vi "IO.vi"() -> ()   [LabVIEW 2020]
uses:
  Global_Variable/Global.vi
  Libraries/S7/S7.lvlib
panel:
  in  "选项卡控件":enum32{"DI", "DO", "伺服"}(tab)
  out "I 1":T1
  out "I 3":T2
  out "I 2":T3
  out "I 0":T4
  out "I 4":T5
  out "I 5":T6
  in  "Q5":T6
  in  "Q4":T7
  in  "Q3":T8
  in  "Q2":T9
  in  "Q1":T10
  in  "Q0":T11
  in  "输入轴旋转手动速度":sgl caption="手动速度" format="%#.3f"
  in  "输入轴旋转-正转":bool
  in  "输入轴旋转-反转":bool
  in  "输入轴旋转绝对位置":sgl caption="绝对位置" format="%#.3f"
  in  "输入轴旋转相对位置":sgl caption="相对位置" format="%#.3f"
  out "输入轴旋转当前位置":sgl caption="当前位置" format="%#.3f"
  in  "输入轴旋转-绝对定位":bool
  in  "输入轴旋转-相对定位":bool
  in  "输入轴移载手动速度":sgl caption="手动速度" format="%#.3f"
  in  "输入轴移载-正转":bool
  in  "输入轴移载-反转":bool
  in  "输入轴移载绝对位置":sgl caption="绝对位置" format="%#.3f"
  in  "输入轴移载相对位置":sgl caption="相对位置" format="%#.3f"
  out "输入轴移载当前位置":sgl caption="当前位置" format="%#.3f"
  in  "输入轴移载-绝对定位":bool
  in  "输入轴移载-相对定位":bool
  in  "工装移载手动速度":sgl caption="手动速度" format="%#.3f"
  in  "工装移载-正转":bool
  in  "工装移载-反转":bool
  in  "工装移载绝对位置":sgl caption="绝对位置" format="%#.3f"
  in  "工装移载相对位置":sgl caption="相对位置" format="%#.3f"
  out "工装移载当前位置":sgl caption="当前位置" format="%#.3f"
  in  "工装移载-绝对定位":bool
  in  "工装移载-相对定位":bool
  out "输入轴旋转状态":bool
  out "输入轴移载状态":bool
  out "工装移载状态":bool
  out "输出轴旋转状态":bool
  out "输入扭矩":sgl format="%#.3f"
  out "输出扭矩(小)":sgl format="%#.3f"
  out "输出扭矩(大)":sgl format="%#.3f"
  out "吸收电流":sgl format="%#.3f"
  # "手动操作"
  # "输入轴旋转伺服"
  # "输入轴移载伺服"
  # "工装移载伺服"
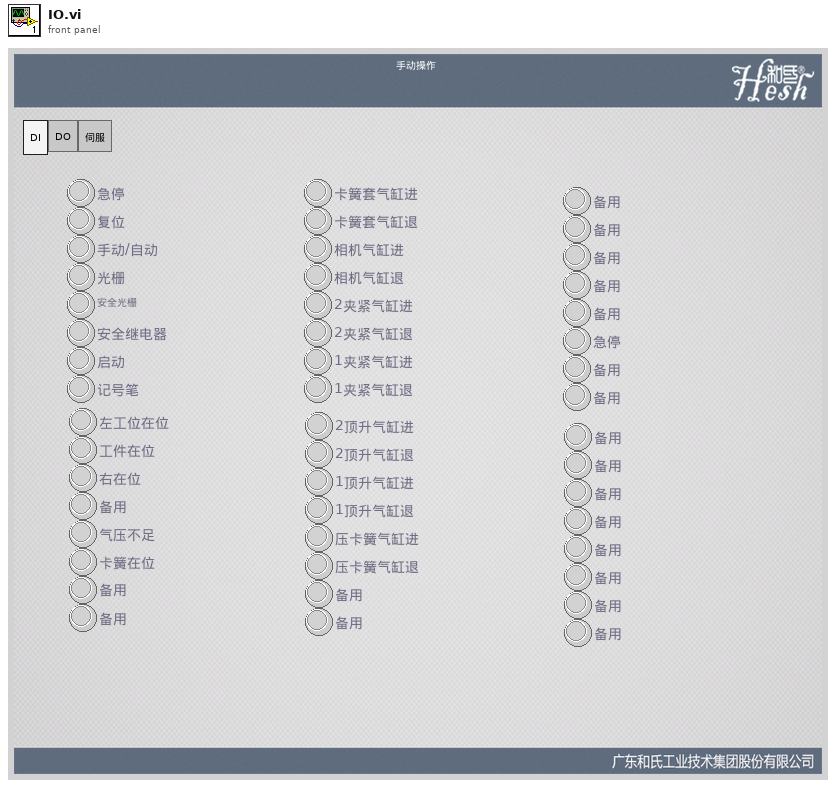
[diagram p1: front panel]
types:
  T1 = cluster{"左工位在位":bool, "工件在位":bool, "右在位":bool, "备用":bool, "气压不足":bool, "卡簧在位":bool, "备用":bool, "备用 ":bool}
  T2 = cluster{"2顶升气缸进":bool, "2顶升气缸退":bool, "1顶升气缸进":bool, "1顶升气缸退":bool, "压卡簧气缸进":bool, "压卡簧气缸退":bool, "备用":bool, "备用":bool}
  T3 = cluster{"卡簧套气缸进":bool, "卡簧套气缸退":bool, "相机气缸进":bool, "相机气缸退":bool, "2夹紧气缸进":bool, "2夹紧气缸退":bool, "1夹紧气缸进":bool, "1夹紧气缸退":bool}
  T4 = cluster{"急停":bool, "复位":bool, "手动/自动":bool, "光栅":bool, "安全光栅":bool, "安全继电器":bool, "启动":bool, "记号笔":bool}
  T5 = cluster{"备用":bool, "备用":bool, "备用":bool, "备用":bool, "备用":bool, "急停":bool, "备用":bool, "备用":bool}
  T6 = cluster{"备用":bool, "备用":bool, "备用":bool, "备用":bool, "备用":bool, "备用":bool, "备用":bool, "备用":bool}
  T7 = cluster{"总气源":bool, "3工位扶正气缸张开":bool, "备用":bool, "备用":bool, "备用":bool, "备用":bool, "备用":bool, "备用":bool}
  T8 = cluster{"2工位扶正气缸张开":bool, "2工位扶正气缸夹紧":bool, "2工位油缸前进":bool, "2工位抬升气缸升":bool, "3工位油缸进":bool, "2工位抬升气缸降":bool, "2工位增压切换":bool, "3工位扶正气缸夹紧":bool}
  T9 = cluster{"1工位轴承上料气缸进":bool, "1工位轴承上料气缸退":bool, "1工位轴承顶升气缸升":bool, "1工位轴承顶升气缸降":bool, "2工位定型气缸进":bool, "2工位定型气缸退":bool, "3工位旋转气缸进":bool, "3工位旋转气缸退":bool}
  T10 = cluster{"OK指示":bool, "NG指示":bool, "/":bool, "/":bool, "/":bool, "/":bool, "/":bool, "/":bool}
  T11 = cluster{"备用":bool, "备用":bool, "备用":bool, "备用":bool, "蜂鸣器":bool, "三色灯黄":bool, "三色灯绿":bool, "三色灯红":bool}
  T12 = cluster{bool, bool, bool, bool, bool, bool, bool, bool}
  T13 = cluster{"[0]":bool, "[1]":bool, "[2]":bool, "[3]":bool, "[4]":bool, "[5]":bool, "[6]":bool, "[7]":bool}
  T14 = typedef "S7.lvlib/Read_Data (Reply Payload)--cluster.ctl" = cluster{"读取成功":bool, "数据":u32[], "Read_Data_error":errorcluster}
  T15 = cluster{"Boolean array[0]":bool, "Boolean array[1]":bool, "Boolean array[2]":bool, "Boolean array[3]":bool, "Boolean array[4]":bool, "Boolean array[5]":bool, "Boolean array[6]":bool, "Boolean array[7]":bool}
  T16 = cluster{"电缸压力":dbl, "电缸位移":sgl, "工装移载位移":sgl, "1":sgl, "输入扭矩":sgl, "大幅":sgl, "输出扭矩(大)":sgl, "大幅度":sgl}
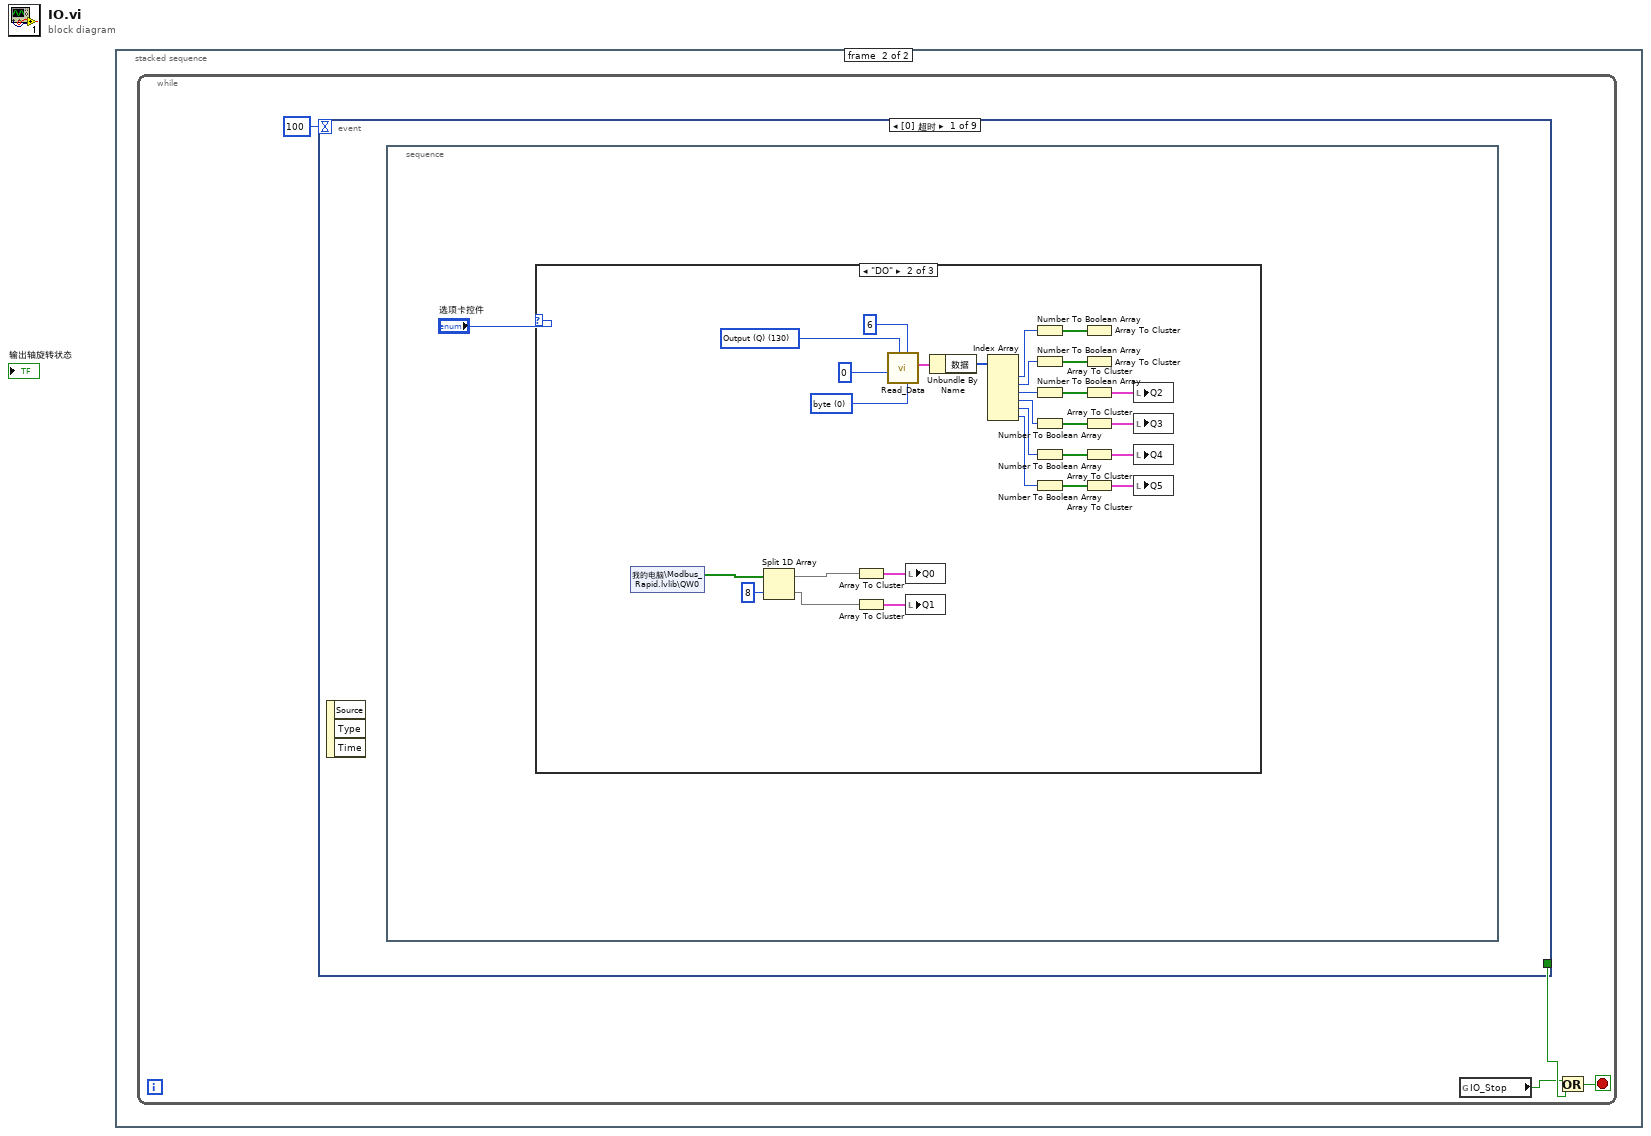
[diagram p0: block diagram]
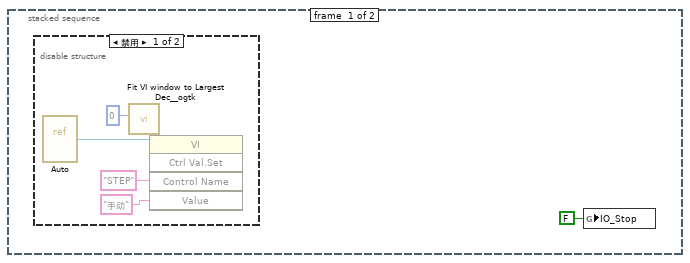
[diagram p2: hidden frame]
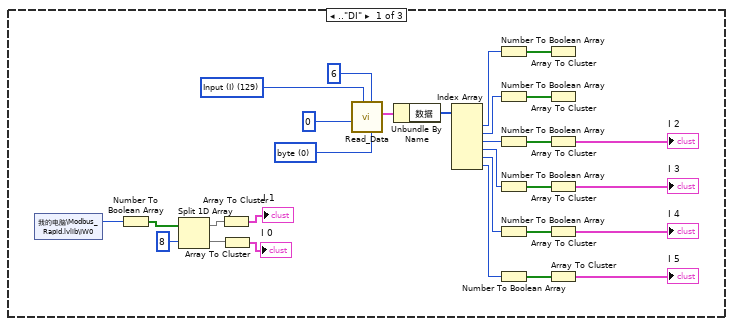
[diagram p4: hidden frame]
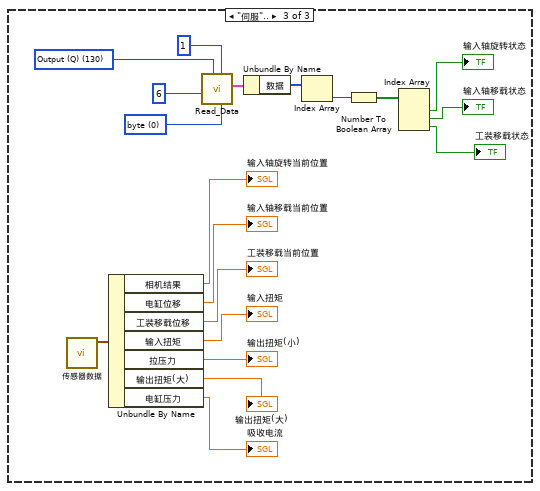
[diagram p5: hidden frame]
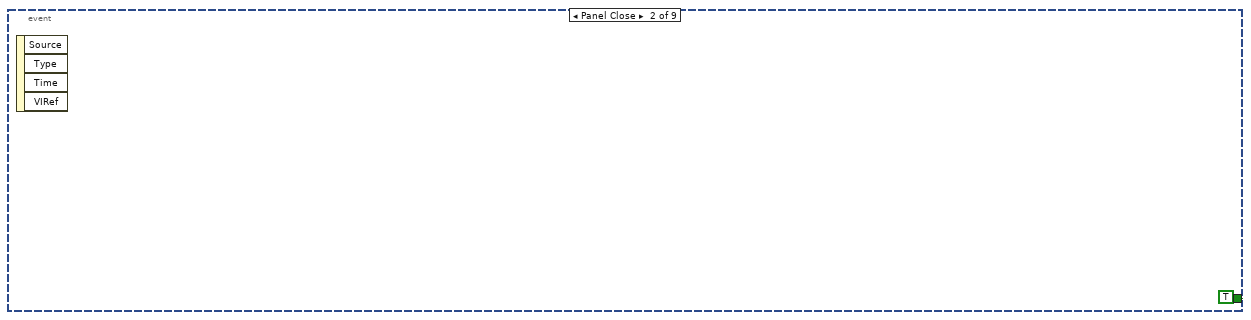
[diagram p6: hidden frame]
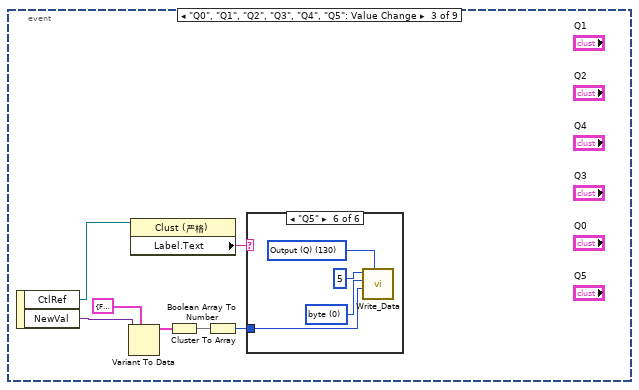
[diagram p7: hidden frame]
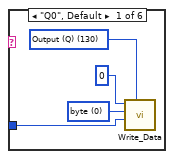
[diagram p8: hidden frame]
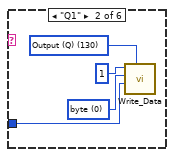
[diagram p9: hidden frame]
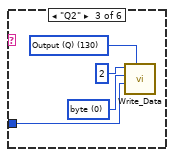
[diagram p10: hidden frame]
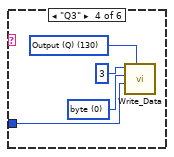
[diagram p11: hidden frame]
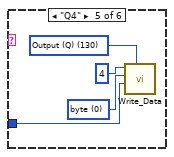
[diagram p12: hidden frame]
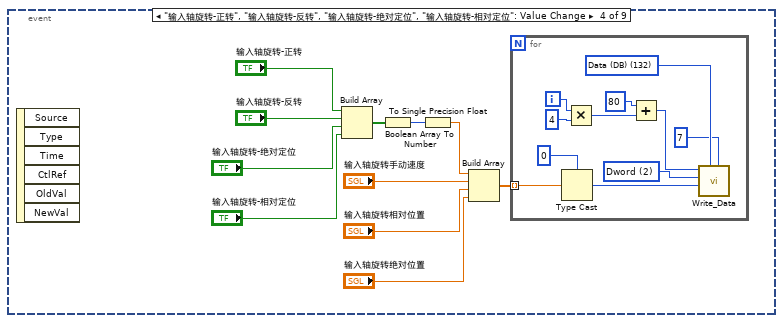
[diagram p13: hidden frame]
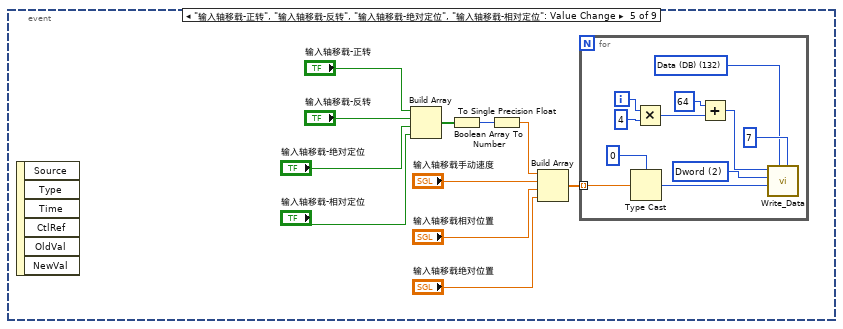
[diagram p14: hidden frame]
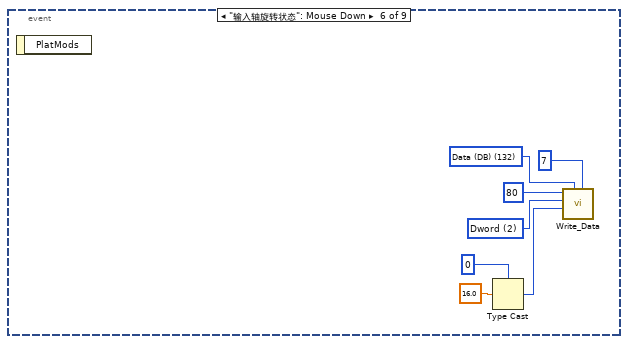
[diagram p15: hidden frame]
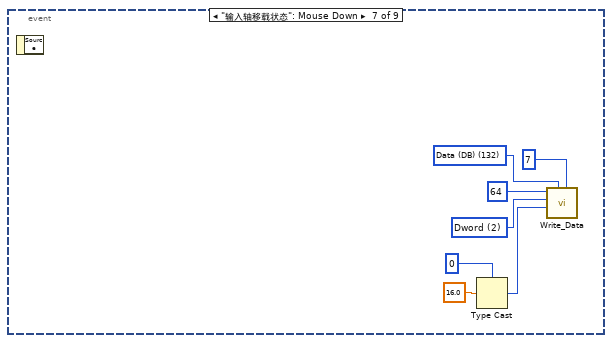
[diagram p16: hidden frame]
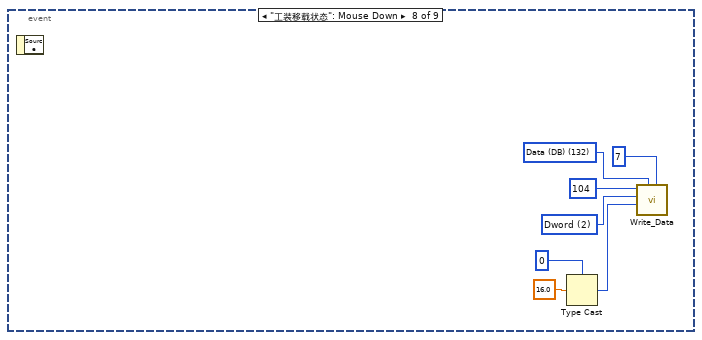
[diagram p17: hidden frame]
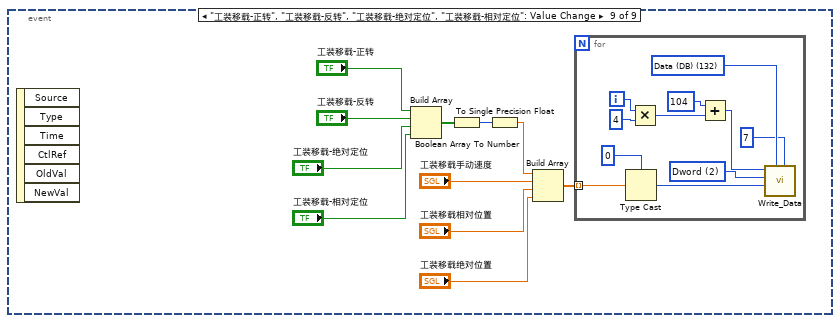
[diagram p18: hidden frame]
diagram:
  n1 = stacked-sequence {
    frame #0 {
      n2 = disable-structure shown="禁用" {
        frame Disabled {
          n3 = vi-ref "Auto.vi"() -> (w4:refnum<vi>)
          n4 = call <userlib>:"Fit VI window to Largest Dec__ogtk.vi"("border spacing (2 px)"=0) -> ()  [unwired: 5 in, 2 out]
          n5 = invoke class="VI" method="Ctrl Val.Set"(reference=w4, "Control Name"="STEP" ("控件名"), "Value"="手动" ("控件名")) -> ()  [unwired: 2 in, 5 out]
        }
        frame Enabled {
        }
      }
      n6 = global write "Global.vi" "IO_Stop"(FALSE ("IO_Stop")) -> ()
    }
    frame #1 {
      n7 = while {
        stop <- w6 stop-if-true
        n8 = event shown="[0] 超时" {
          selector: _ -> [_ _ _ _ _ _ _ _ _]
          dyn-events: _ -> [_ _ _ _ _ _ _ _ _]
          timeout: 100 -> [_ _ _ _ _ _ _ _ _]
          tunnel: [_ TRUE _ _ _ _ _ _ _] -> w8
          event Timeout {
            n9 = event-data() -> ()  [unwired: 1 in, 3 out]
            n10 = stacked-sequence {
              frame #0 {
                n11 = case shown="\"DO\"" "选项卡控件" {
                  frame .."DI" {
                    w21 = u16 0 items=["byte", "word", "Dword"] ("数据类型")
                    w19 = u8 129 items=["I/O (P)"=128, "Input (I)"=129, "Output (Q)"=130, "Bit Memory (M)"=131, "Data (DB)"=132, "Instance Data (DI)"=133, "Local Data (L)"=134, "Predecessor Local Data (VL)"=135] ("寄存器类型")
                    n12 = shared-variable "我的电脑\\Modbus_Rapid.lvlib\\IW0"() -> (w17:u16)  [unwired: 1 in, 1 out]
                    n13 = Number To Boolean Array(number=w17) -> (Boolean array=w16:bool[])
                    n14 = Split 1D Array(array=w16, index=8 ("索引")) -> (first subarray=w15:bool[], second subarray=w13:bool[])
                    n15 = Array To Cluster(array=w15) -> (cluster=→"I 1":T13)
                    n16 = Array To Cluster(array=w13) -> (cluster=→"I 0":T13)
                    n17 = call "Read_Data.vi"("数据类型"=w21, "读取长度"=u16 6, "寄存器类型"=w19, "起始地址"=u32 0) -> ("Reply Payload"=w23:T14)  [unwired: 5 in, 2 out]
                    n18 = Unbundle By Name(w23) -> ("数据"=w22:u32[])
                    n19 = Index Array(array=w22) -> (element #1=w35:u32, element #2=w37:u32, element #3=w36:u32, element #4=w32:u32, element #5=w31:u32, element #6=w30:u32)  [unwired: 6 in]
                    n20 = Number To Boolean Array(number=w35) -> (Boolean array=w34:bool[])
                    n21 = Number To Boolean Array(number=w37) -> (Boolean array=w33:bool[])
                    n22 = Number To Boolean Array(number=w36) -> (Boolean array=w29:bool[])
                    n23 = Number To Boolean Array(number=w32) -> (Boolean array=w27:bool[])
                    n24 = Number To Boolean Array(number=w31) -> (Boolean array=w25:bool[])
                    n25 = Number To Boolean Array(number=w30) -> (Boolean array=w24:bool[])
                    n26 = Array To Cluster(array=w34) -> ()  [unwired: 1 out]
                    n27 = Array To Cluster(array=w33) -> ()  [unwired: 1 out]
                    n28 = Array To Cluster(array=w29) -> (cluster=→"I 2":T15)
                    n29 = Array To Cluster(array=w27) -> (cluster=→"I 3":T15)
                    n30 = Array To Cluster(array=w25) -> (cluster=→"I 4":T15)
                    n31 = Array To Cluster(array=w24) -> (cluster=→"I 5":T15)
                  }
                  frame "DO" {
                    w49 = u16 0 items=["byte", "word", "Dword"] ("数据类型")
                    w47 = u8 130 items=["I/O (P)"=128, "Input (I)"=129, "Output (Q)"=130, "Bit Memory (M)"=131, "Data (DB)"=132, "Instance Data (DI)"=133, "Local Data (L)"=134, "Predecessor Local Data (VL)"=135] ("寄存器类型")
                    n32 = shared-variable "我的电脑\\Modbus_Rapid.lvlib\\QW0"() -> (w40:bool[])  [unwired: 1 in, 1 out]
                    n33 = Split 1D Array(array=w40, index=8 ("索引")) -> (first subarray=w42:bool[], second subarray=w41:bool[])
                    n34 = Array To Cluster(array=w42) -> (cluster=w44:T13)
                    n35 = Array To Cluster(array=w41) -> (cluster=w43:T13)
                    n36 = call "Read_Data.vi"("数据类型"=w49, "读取长度"=u16 6, "寄存器类型"=w47, "起始地址"=u32 0) -> ("Reply Payload"=w66:T14)  [unwired: 5 in, 2 out]
                    n37 = local write "Q0"(w44) -> ()
                    n38 = local write "Q1"(w43) -> ()
                    n39 = Unbundle By Name(w66) -> ("数据"=w67:u32[])
                    n40 = Index Array(array=w67) -> (element #1=w57:u32, element #2=w59:u32, element #3=w58:u32, element #4=w56:u32, element #5=w55:u32, element #6=w54:u32)  [unwired: 6 in]
                    n41 = Number To Boolean Array(number=w57) -> (Boolean array=w60:bool[])
                    n42 = Number To Boolean Array(number=w59) -> (Boolean array=w61:bool[])
                    n43 = Number To Boolean Array(number=w58) -> (Boolean array=w62:bool[])
                    n44 = Number To Boolean Array(number=w56) -> (Boolean array=w63:bool[])
                    n45 = Number To Boolean Array(number=w55) -> (Boolean array=w64:bool[])
                    n46 = Number To Boolean Array(number=w54) -> (Boolean array=w65:bool[])
                    n47 = Array To Cluster(array=w60) -> ()  [unwired: 1 out]
                    n48 = Array To Cluster(array=w61) -> ()  [unwired: 1 out]
                    n49 = Array To Cluster(array=w62) -> (cluster=w52:T15)
                    n50 = Array To Cluster(array=w63) -> (cluster=w53:T15)
                    n51 = Array To Cluster(array=w64) -> (cluster=w51:T15)
                    n52 = Array To Cluster(array=w65) -> (cluster=w50:T15)
                    n53 = local write "Q2"(w52) -> ()
                    n54 = local write "Q3"(w53) -> ()
                    n55 = local write "Q4"(w51) -> ()
                    n56 = local write "Q5"(w50) -> ()
                  }
                  frame "伺服".. {
                    w79 = u16 0 items=["byte", "word", "Dword"] ("数据类型")
                    w77 = u8 130 items=["I/O (P)"=128, "Input (I)"=129, "Output (Q)"=130, "Bit Memory (M)"=131, "Data (DB)"=132, "Instance Data (DI)"=133, "Local Data (L)"=134, "Predecessor Local Data (VL)"=135] ("寄存器类型")
                    n57 = call "传感器数据.vi"() -> ("传感器读数"=w71:T16)  [unwired: 11 in]
                    n58 = Unbundle By Name(w71) -> ("相机结果"=→"输入轴旋转当前位置":dbl, "电缸位移"=→"输入轴移载当前位置":sgl, "工装移载位移"=→"工装移载当前位置":sgl, "输入扭矩"=→"输入扭矩":sgl, "拉压力"=→"输出扭矩(小)":sgl, "输出扭矩(大)"=→"输出扭矩(大)":sgl, "电缸压力"=→"吸收电流":dbl)
                    n59 = call "Read_Data.vi"("数据类型"=w79, "读取长度"=u16 1, "寄存器类型"=w77, "起始地址"=u32 6) -> ("Reply Payload"=w80:T14)  [unwired: 5 in, 2 out]
                    n60 = Unbundle By Name(w80) -> ("数据"=w81:u32[])
                    n61 = Index Array(array=w81) -> (element=w86:u32)  [unwired: 1 in]
                    n62 = Number To Boolean Array(number=w86) -> (Boolean array=w83:bool[])
                    n63 = Index Array(array=w83) -> (element #1=→"输入轴旋转状态":bool, element #2=→"输入轴移载状态":bool, element #3=→"工装移载状态":bool)  [unwired: 3 in]
                  }
                }
              }
            }
          }
          event Panel Close {
            n64 = event-data() -> ()  [unwired: 1 in, 4 out]
          }
          event "Q0", "Q1", "Q2", "Q3", "Q4", "Q5": Value Change {
            n65 = event-data() -> ("CtlRef"=w89:refnum<vi>, "NewVal"=w93:variant)  [unwired: 1 in]
            n66 = Variant To Data(type=T12 {FALSE, FALSE, FALSE, FALSE, FALSE, FALSE, FALSE, FALSE}, Variant=w93) -> (data=w92:T12)  [unwired: 1 in, 1 out]
            n67 = property class="Clust (严格)"(reference=w89) -> ("Label.Text"=w88:string)  [unwired: 1 in, 2 out]
            n68 = Cluster To Array(cluster=w92) -> (array=w91:bool[])
            n69 = Boolean Array To Number(Boolean array=w91) -> (number=w90:u32)
            n70 = case shown="\"Q5\"" w88 {
              tunnel: w90 -> [w98 w102 w106 w110 w114 w118]
              frame "Q0", Default {
                w96 = u16 0 items=["byte", "word", "Dword"] ("数据类型")
                w97 = u8 130 items=["I/O (P)"=128, "Input (I)"=129, "Output (Q)"=130, "Bit Memory (M)"=131, "Data (DB)"=132, "Instance Data (DI)"=133, "Local Data (L)"=134, "Predecessor Local Data (VL)"=135] ("寄存器类型")
                n71 = call "Write_Data.vi"("寄存器类型"=w97, "写入数据"=w98, "数据类型"=w96, "写入地址"=u32 0) -> ()  [unwired: 5 in, 3 out]
              }
              frame "Q1" {
                w100 = u16 0 items=["byte", "word", "Dword"] ("数据类型")
                w101 = u8 130 items=["I/O (P)"=128, "Input (I)"=129, "Output (Q)"=130, "Bit Memory (M)"=131, "Data (DB)"=132, "Instance Data (DI)"=133, "Local Data (L)"=134, "Predecessor Local Data (VL)"=135] ("寄存器类型")
                n72 = call "Write_Data.vi"("寄存器类型"=w101, "写入数据"=w102, "数据类型"=w100, "写入地址"=u32 1) -> ()  [unwired: 5 in, 3 out]
              }
              frame "Q2" {
                w104 = u16 0 items=["byte", "word", "Dword"] ("数据类型")
                w105 = u8 130 items=["I/O (P)"=128, "Input (I)"=129, "Output (Q)"=130, "Bit Memory (M)"=131, "Data (DB)"=132, "Instance Data (DI)"=133, "Local Data (L)"=134, "Predecessor Local Data (VL)"=135] ("寄存器类型")
                n73 = call "Write_Data.vi"("寄存器类型"=w105, "写入数据"=w106, "数据类型"=w104, "写入地址"=u32 2) -> ()  [unwired: 5 in, 3 out]
              }
              frame "Q3" {
                w108 = u16 0 items=["byte", "word", "Dword"] ("数据类型")
                w109 = u8 130 items=["I/O (P)"=128, "Input (I)"=129, "Output (Q)"=130, "Bit Memory (M)"=131, "Data (DB)"=132, "Instance Data (DI)"=133, "Local Data (L)"=134, "Predecessor Local Data (VL)"=135] ("寄存器类型")
                n74 = call "Write_Data.vi"("寄存器类型"=w109, "写入数据"=w110, "数据类型"=w108, "写入地址"=u32 3) -> ()  [unwired: 5 in, 3 out]
              }
              frame "Q4" {
                w112 = u16 0 items=["byte", "word", "Dword"] ("数据类型")
                w113 = u8 130 items=["I/O (P)"=128, "Input (I)"=129, "Output (Q)"=130, "Bit Memory (M)"=131, "Data (DB)"=132, "Instance Data (DI)"=133, "Local Data (L)"=134, "Predecessor Local Data (VL)"=135] ("寄存器类型")
                n75 = call "Write_Data.vi"("寄存器类型"=w113, "写入数据"=w114, "数据类型"=w112, "写入地址"=u32 4) -> ()  [unwired: 5 in, 3 out]
              }
              frame "Q5" {
                w116 = u16 0 items=["byte", "word", "Dword"] ("数据类型")
                w117 = u8 130 items=["I/O (P)"=128, "Input (I)"=129, "Output (Q)"=130, "Bit Memory (M)"=131, "Data (DB)"=132, "Instance Data (DI)"=133, "Local Data (L)"=134, "Predecessor Local Data (VL)"=135] ("寄存器类型")
                n76 = call "Write_Data.vi"("寄存器类型"=w117, "写入数据"=w118, "数据类型"=w116, "写入地址"=u32 5) -> ()  [unwired: 5 in, 3 out]
              }
            }
          }
          event "输入轴旋转-正转", "输入轴旋转-反转", "输入轴旋转-绝对定位", "输入轴旋转-相对定位": Value Change {
            n77 = event-data() -> ()  [unwired: 1 in, 6 out]
            n78 = Build Array("输入轴旋转-正转", "输入轴旋转-反转", "输入轴旋转-绝对定位", "输入轴旋转-相对定位") -> (w128:bool[])
            n79 = Boolean Array To Number(Boolean array=w128) -> (number=w127:u32)
            n80 = To Single Precision Float(number=w127) -> (single precision float=w129:sgl)
            n81 = Build Array(w129, "输入轴旋转手动速度", "输入轴旋转相对位置", "输入轴旋转绝对位置") -> (w126:sgl[])
            n82 = for {
              tunnel: w126 -> [w135] mode=indexing
              i -> [w132]
              w137 = u16 2 items=["byte", "word", "Dword"] ("数据类型")
              w140 = u8 132 items=["I/O (P)"=128, "Input (I)"=129, "Output (Q)"=130, "Bit Memory (M)"=131, "Data (DB)"=132, "Instance Data (DI)"=133, "Local Data (L)"=134, "Predecessor Local Data (VL)"=135] ("寄存器类型")
              n83 = Type Cast(type=u32 0, x=w135) -> (*(type *) &x=w134:u32)
              n84 = Multiply(x=w132, y=u32 4) -> (x*y=w131:u32)
              n85 = Add(x=u32 80 ("写入地址"), y=w131) -> (x+y=w130:u32)
              n86 = call "Write_Data.vi"("DB #"=u16 7, "寄存器类型"=w140, "写入数据"=w134, "数据类型"=w137, "写入地址"=w130) -> ()  [unwired: 4 in, 3 out]
            }
          }
          event "输入轴移载-正转", "输入轴移载-反转", "输入轴移载-绝对定位", "输入轴移载-相对定位": Value Change {
            n87 = event-data() -> ()  [unwired: 1 in, 6 out]
            n88 = Build Array("输入轴移载-正转", "输入轴移载-反转", "输入轴移载-绝对定位", "输入轴移载-相对定位") -> (w150:bool[])
            n89 = Boolean Array To Number(Boolean array=w150) -> (number=w149:u32)
            n90 = To Single Precision Float(number=w149) -> (single precision float=w151:sgl)
            n91 = Build Array(w151, "输入轴移载手动速度", "输入轴移载相对位置", "输入轴移载绝对位置") -> (w148:sgl[])
            n92 = for {
              tunnel: w148 -> [w160] mode=indexing
              i -> [w158]
              w153 = u16 2 items=["byte", "word", "Dword"] ("数据类型")
              w155 = u8 132 items=["I/O (P)"=128, "Input (I)"=129, "Output (Q)"=130, "Bit Memory (M)"=131, "Data (DB)"=132, "Instance Data (DI)"=133, "Local Data (L)"=134, "Predecessor Local Data (VL)"=135] ("寄存器类型")
              n93 = Type Cast(type=u32 0, x=w160) -> (*(type *) &x=w152:u32)
              n94 = Multiply(x=w158, y=u32 4) -> (x*y=w157:u32)
              n95 = Add(x=u32 64 ("写入地址"), y=w157) -> (x+y=w154:u32)
              n96 = call "Write_Data.vi"("DB #"=u16 7, "寄存器类型"=w155, "写入数据"=w152, "数据类型"=w153, "写入地址"=w154) -> ()  [unwired: 4 in, 3 out]
            }
          }
          event "输入轴旋转状态": Mouse Down {
            w165 = u16 2 items=["byte", "word", "Dword"] ("数据类型")
            w167 = u8 132 items=["I/O (P)"=128, "Input (I)"=129, "Output (Q)"=130, "Bit Memory (M)"=131, "Data (DB)"=132, "Instance Data (DI)"=133, "Local Data (L)"=134, "Predecessor Local Data (VL)"=135] ("寄存器类型")
            n97 = event-data() -> ()  [unwired: 1 in, 1 out]
            n98 = Type Cast(type=u32 0, x=sgl 16.0) -> (*(type *) &x=w169:u32)
            n99 = call "Write_Data.vi"("DB #"=u16 7, "寄存器类型"=w167, "写入数据"=w169, "数据类型"=w165, "写入地址"=u32 80) -> ()  [unwired: 4 in, 3 out]
          }
          event "输入轴移载状态": Mouse Down {
            w170 = u16 2 items=["byte", "word", "Dword"] ("数据类型")
            w173 = u8 132 items=["I/O (P)"=128, "Input (I)"=129, "Output (Q)"=130, "Bit Memory (M)"=131, "Data (DB)"=132, "Instance Data (DI)"=133, "Local Data (L)"=134, "Predecessor Local Data (VL)"=135] ("寄存器类型")
            n100 = event-data() -> ()  [unwired: 1 in, 1 out]
            n101 = Type Cast(type=u32 0, x=sgl 16.0) -> (*(type *) &x=w176:u32)
            n102 = call "Write_Data.vi"("DB #"=u16 7, "寄存器类型"=w173, "写入数据"=w176, "数据类型"=w170, "写入地址"=u32 64) -> ()  [unwired: 4 in, 3 out]
          }
          event "工装移载状态": Mouse Down {
            w177 = u16 2 items=["byte", "word", "Dword"] ("数据类型")
            w180 = u8 132 items=["I/O (P)"=128, "Input (I)"=129, "Output (Q)"=130, "Bit Memory (M)"=131, "Data (DB)"=132, "Instance Data (DI)"=133, "Local Data (L)"=134, "Predecessor Local Data (VL)"=135] ("寄存器类型")
            n103 = event-data() -> ()  [unwired: 1 in, 1 out]
            n104 = Type Cast(type=u32 0, x=sgl 16.0) -> (*(type *) &x=w183:u32)
            n105 = call "Write_Data.vi"("DB #"=u16 7, "寄存器类型"=w180, "写入数据"=w183, "数据类型"=w177, "写入地址"=u32 104) -> ()  [unwired: 4 in, 3 out]
          }
          event "工装移载-正转", "工装移载-反转", "工装移载-绝对定位", "工装移载-相对定位": Value Change {
            n106 = event-data() -> ()  [unwired: 1 in, 6 out]
            n107 = Build Array("工装移载-正转", "工装移载-反转", "工装移载-绝对定位", "工装移载-相对定位") -> (w190:bool[])
            n108 = Boolean Array To Number(Boolean array=w190) -> (number=w189:u32)
            n109 = To Single Precision Float(number=w189) -> (single precision float=w188:sgl)
            n110 = Build Array(w188, "工装移载手动速度", "工装移载相对位置", "工装移载绝对位置") -> (w186:sgl[])
            n111 = for {
              tunnel: w186 -> [w200] mode=indexing
              i -> [w197]
              w202 = u16 2 items=["byte", "word", "Dword"] ("数据类型")
              w205 = u8 132 items=["I/O (P)"=128, "Input (I)"=129, "Output (Q)"=130, "Bit Memory (M)"=131, "Data (DB)"=132, "Instance Data (DI)"=133, "Local Data (L)"=134, "Predecessor Local Data (VL)"=135] ("寄存器类型")
              n112 = Type Cast(type=u32 0, x=w200) -> (*(type *) &x=w199:u32)
              n113 = Multiply(x=w197, y=u32 4) -> (x*y=w196:u32)
              n114 = Add(x=u32 104 ("写入地址"), y=w196) -> (x+y=w195:u32)
              n115 = call "Write_Data.vi"("DB #"=u16 7, "寄存器类型"=w205, "写入数据"=w199, "数据类型"=w202, "写入地址"=w195) -> ()  [unwired: 4 in, 3 out]
            }
          }
        }
        n116 = global read "Global.vi" "IO_Stop"() -> (w7:bool)
        n117 = Or(x=w7, y=w8) -> (x .or. y?=w6:bool)
      }
    }
  }
